vi "Cleanup.vi"(8 "error in (no error)":errorcluster, 11 "picoG in":refnum<class "picoG.lvclass">) -> (0 "error out":errorcluster)   [LabVIEW 2020, in "PicoG-App.lvlib" / "picoG.lvclass"]
uses:
  picoG.lvclass
  picoG.lvclass/picoG.ctl
  <vilib>/IlluminatedG/IG OOPanel/OOPanel/Manager/Manager.lvclass
  App Watcher/App Watcher.lvclass
  Builds/picoG/ppl/PicoG-Core.lvlibp/PicoG-Processor/PicoG-Core/PlatformManager/PlatformManager.lvclass
  Device/Device.lvclass
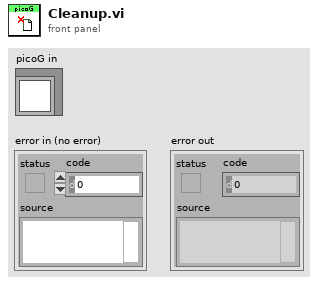
[diagram p1: front panel]
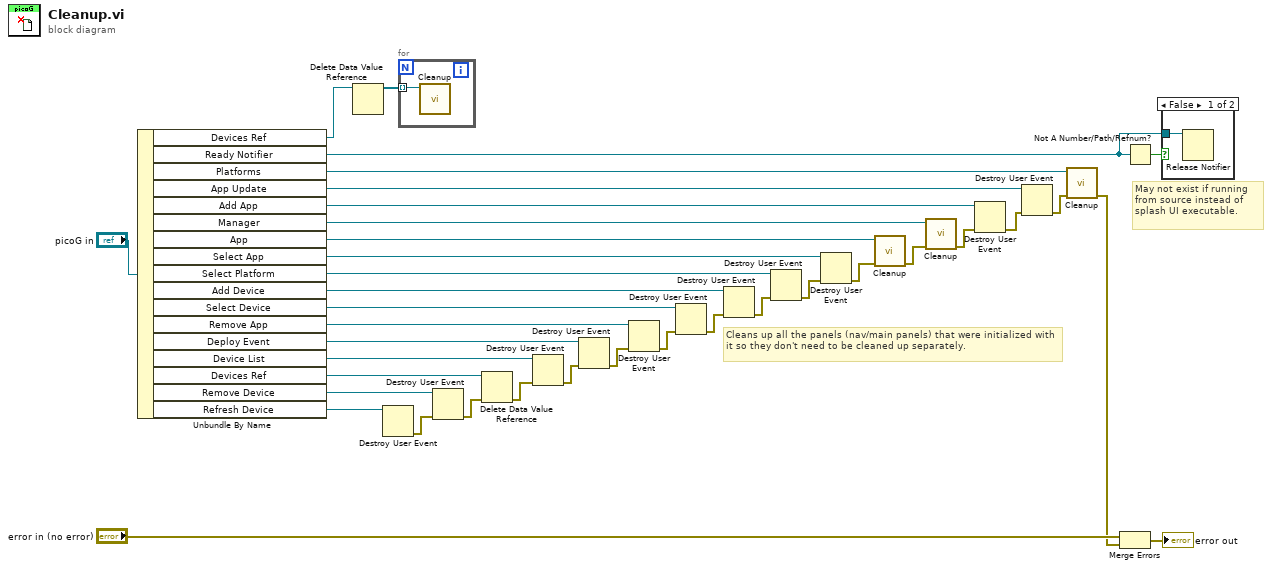
[diagram p0: block diagram]
diagram:
  # "May not exist if running from source instead of splash UI executable."
  # "Cleans up all the panels (nav/main panels) that were initialized with it so they don't need to be cleaned up separately."
  n1 = Unbundle By Name("picoG in") -> ("Devices Ref"=w4:refnum<data-value>, "Ready Notifier"=w27:refnum<notifier>, "Platforms"=w30:refnum<class "PlatformManager.lvclass">, "App Update"=w25:refnum<user-event>, "Add App"=w34:refnum<user-event>, "Manager"=w35:refnum<class "Manager.lvclass">, "App"=w32:refnum<class "App Watcher.lvclass">, "Select App"=w22:refnum<user-event>, "Select Platform"=w23:refnum<user-event>, "Add Device"=w18:refnum<user-event>, "Select Device"=w16:refnum<user-event>, "Remove App"=w14:refnum<user-event>, "Deploy Event"=w11:refnum<user-event>, "Device List"=w9:refnum<user-event>, "Devices Ref"=w8:refnum<data-value>, "Remove Device"=w6:refnum<user-event>, "Refresh Device"=w1:refnum<user-event>)
  n2 = Delete Data Value Reference(data value reference=w4) -> (data value=w3:refnum<class "Device.lvclass">[])  [unwired: 1 in, 1 out]
  n3 = Destroy User Event(user event=w1) -> (error out=w2:errorcluster)  [unwired: 1 in]
  n4 = for {
    tunnel: w3 -> [w38] mode=indexing
    n5 = call <vilib>:"Cleanup.vi"("Device in"=w38) -> ()  [unwired: 10 in, 1 out]
  }
  n6 = Destroy User Event(user event=w6, error in=w2) -> (error out=w5:errorcluster)
  n7 = Delete Data Value Reference(data value reference=w8, error in=w5) -> (error out=w7:errorcluster)  [unwired: 1 out]
  n8 = Destroy User Event(user event=w9, error in=w7) -> (error out=w10:errorcluster)
  n9 = Destroy User Event(user event=w11, error in=w10) -> (error out=w12:errorcluster)
  n10 = Destroy User Event(user event=w14, error in=w12) -> (error out=w13:errorcluster)
  n11 = Destroy User Event(user event=w16, error in=w13) -> (error out=w15:errorcluster)
  n12 = Destroy User Event(user event=w18, error in=w15) -> (error out=w17:errorcluster)
  n13 = Destroy User Event(user event=w23, error in=w17) -> (error out=w21:errorcluster)
  n14 = Destroy User Event(user event=w22, error in=w21) -> (error out=w20:errorcluster)
  n15 = call <vilib>:"Cleanup.vi"("error in (no error)"=w20, "App Watcher in"=w32) -> ("error out"=w31:errorcluster)  [unwired: 9 in]
  n16 = call <vilib>:"Cleanup.vi"("error in (no error)"=w31, "Manager in"=w35) -> ("error out"=w33:errorcluster)  [unwired: 7 in, 2 out]
  n17 = Destroy User Event(user event=w34, error in=w33) -> (error out=w19:errorcluster)
  n18 = Destroy User Event(user event=w25, error in=w19) -> (error out=w24:errorcluster)
  n19 = call <vilib>:"Cleanup.vi"("error in (no error)"=w24, "PlatformManager in"=w30) -> ("error out"=w28:errorcluster)  [unwired: 9 in]
  n20 = Merge Errors("error in (no error)", w28) -> (→"error out":errorcluster)
  n21 = Not A Number/Path/Refnum?(number/path/refnum=w27) -> (NaN/Path/Refnum?=w26:bool)
  n22 = case shown="False" w26 {
    tunnel: w27 -> [w39 _]
    frame False {
      n23 = Release Notifier(notifier=w39) -> ()  [unwired: 2 in, 3 out]
    }
    frame True {
    }
  }
